vi "runAnalysis.vi"(8 "error in (no error)":errorcluster, 10 "ImageAnalyser":refnum<class "ImageAnalyser.lvclass">, 11 "ImageStreamViewer in":refnum<class "ImageStreamViewer.lvclass">) -> (0 "error out":errorcluster, 3 "ImageStreamViewer out":refnum<class "ImageStreamViewer.lvclass">)   [LabVIEW 2011, in "Views.lvlib" / "Camera.lvlib" / "ImageStreamViewer.lvclass"]
uses:
  ImageStreamViewer.lvclass
  Tools/ImageProcessor/ImageAnalyser/ImageAnalyser.lvclass
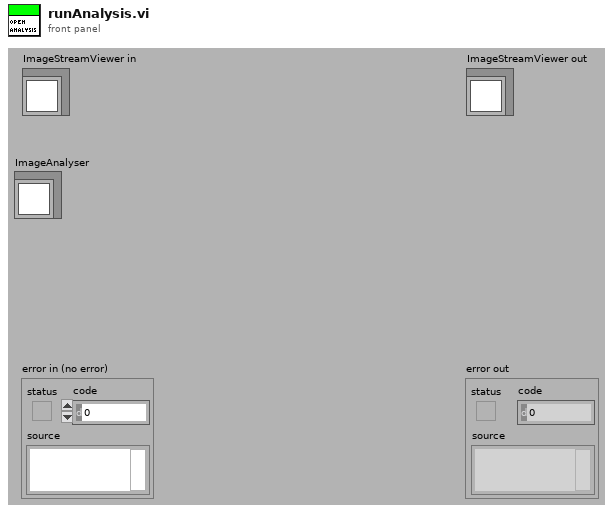
[diagram p1: front panel]
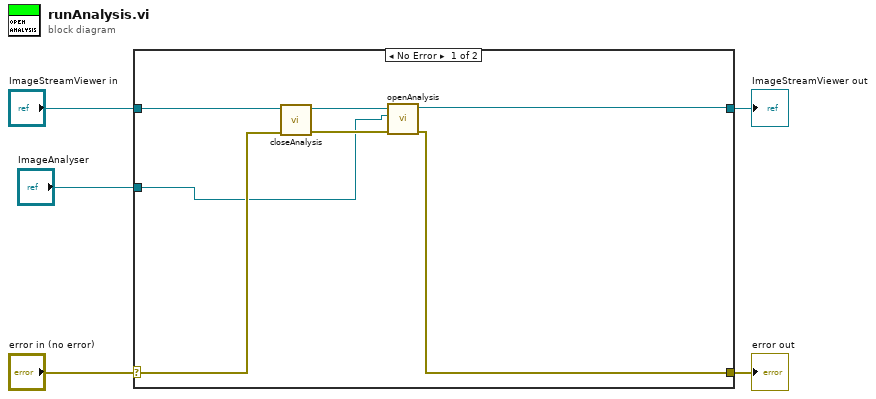
[diagram p0: block diagram]
diagram:
  n1 = case shown="No Error" "error in (no error)" {
    selector: "error in (no error)" -> [w7 w14]
    tunnel: [w11 w14] -> w4
    tunnel: [w12 w13] -> w2
    tunnel: "ImageStreamViewer in" -> [w10 w13]
    tunnel: "ImageAnalyser" -> [w6 _]
    frame No Error {
      n2 = call "closeAnalysis.vi"("error in (no error)"=w7, "ImageStreamViewer in"=w10) -> ("error out"=w8:errorcluster, "ImageStreamViewer out"=w9:refnum<class "ImageStreamViewer.lvclass">)  [unwired: 8 in]
      n3 = call "openAnalysis.vi"("error in (no error)"=w8, "ImageAnalyser"=w6, "ImageStreamViewer in"=w9) -> ("error out"=w11:errorcluster, "ImageStreamViewer out"=w12:refnum<class "ImageStreamViewer.lvclass">)  [unwired: 7 in]
    }
    frame Error {
    }
  }
  "error out" <- w4
  "ImageStreamViewer out" <- w2
